vi "CRYOne Quick Lunch Menu.vi"() -> ()   [LabVIEW 2013]
uses:
  CRYMainGlobal.vi
  CRYWindow/SubVI/CRYMain Sub Window Global.vi
panel:
  out "Arrow2":bool
  out "Arrow1":bool
  out "MarkImage":bool
  in  "Show Dialog Prompt":bool caption="Do not show this dialog again"
  out "bReturn":bool
  in  "Calibrate Microphone":bool caption="OK"
  in  "Setup Test":bool caption="OK"
  in  "Self Test":bool caption="OK"
  in  "stop":bool
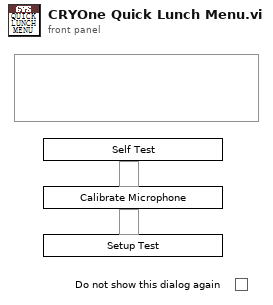
[diagram p1: front panel]
types:
  T1 = enum32{"Invalid", "Standard", "Closed", "Hidden", "Minimized", "Maximized"}
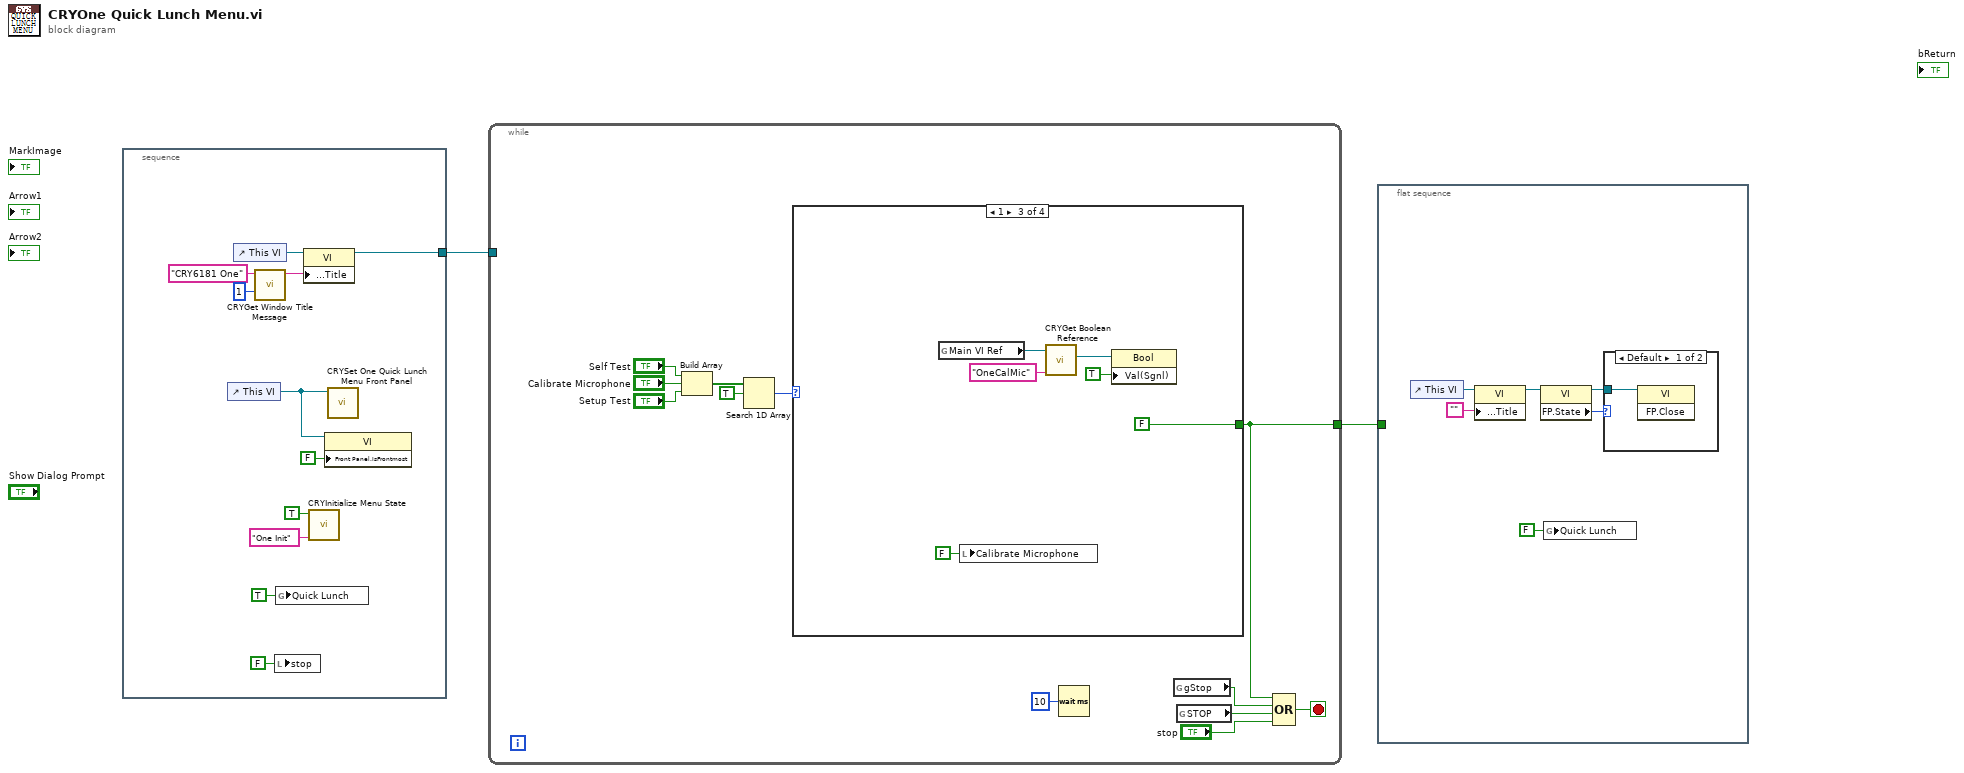
[diagram p0: block diagram]
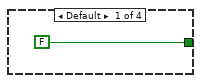
[diagram p3: hidden frame]
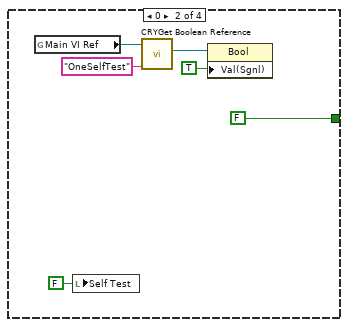
[diagram p4: hidden frame]
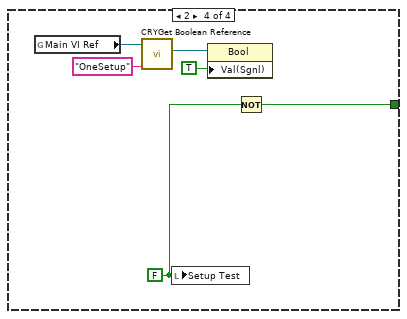
[diagram p5: hidden frame]
diagram:
  n1 = stacked-sequence {
    tunnel: [w6] -> w1
    frame #0 {
      n2 = control-ref of="This VI"() -> (w8:refnum<vi>)
      n3 = control-ref of="This VI"() -> (w11:refnum<vi>)
      n4 = call "CRYGet Window Title Message.vi"("No"=1 ("Error No"), "Kind"="CRY6181 One") -> ("Multibyte String"=w10:string)  [unwired: 4 in, 5 out]
      n5 = local write "stop"(FALSE ("stop")) -> ()
      n6 = global write "CRYMainGlobal.vi" "Quick Lunch"(TRUE ("Quick Lunch")) -> ()
      n7 = property class="VI"(reference=w11, "Front Panel.Title"=w10) -> (reference out=w6:refnum<vi>)  [unwired: 1 in, 1 out]
      n8 = call "CRYInitialize Menu State.vi"("sAction"="One Init", "Is Disable?"=TRUE) -> ()  [unwired: 10 out]
      n9 = property class="VI"(reference=w8, "Front Panel.IsFrontmost"=FALSE ("Front Panel Window:Is Frontmost")) -> ()  [unwired: 1 in, 2 out]
      n10 = call "CRYSet One Quick Lunch Menu Front Panel.vi"("Vi Ref In"=w8) -> ()  [unwired: 10 in, 1 out]
    }
  }
  n11 = while {
    tunnel: [w15] -> w2
    tunnel: w1 -> [_]
    stop <- w14 stop-if-true
    n12 = Build Array("Self Test", "Calibrate Microphone", "Setup Test") -> (w21:bool[])
    n13 = Search 1D Array(1D array=w21, element=TRUE) -> (index of element=w19:i32)  [unwired: 1 in]
    n14 = case shown="1" w19 {
      tunnel: [FALSE FALSE FALSE w43] -> w15
      frame Default {
      }
      frame 0 {
        n15 = global read "CRYMain Sub Window Global.vi" "Main VI Ref"() -> (w30:refnum<vi>)
        n16 = local write "Self Test"(FALSE ("Self Test")) -> ()
        n17 = call "CRYGet Boolean Reference.vi"("Label Name"="OneSelfTest", "VI Refnum"=w30) -> ("Boolean Ref"=w28:refnum<vi>)  [unwired: 7 in, 2 out]
        n18 = property class="Bool"(reference=w28, "Val(Sgnl)"=TRUE) -> ()  [unwired: 1 in, 2 out]
      }
      frame 1 {
        n19 = global read "CRYMain Sub Window Global.vi" "Main VI Ref"() -> (w37:refnum<vi>)
        n20 = local write "Calibrate Microphone"(FALSE ("Calibrate Microphone")) -> ()
        n21 = call "CRYGet Boolean Reference.vi"("Label Name"="OneCalMic", "VI Refnum"=w37) -> ("Boolean Ref"=w35:refnum<vi>)  [unwired: 7 in, 2 out]
        n22 = property class="Bool"(reference=w35, "Val(Sgnl)"=TRUE) -> ()  [unwired: 1 in, 2 out]
      }
      frame 2 {
        w44 = FALSE ("Setup Test")
        n23 = global read "CRYMain Sub Window Global.vi" "Main VI Ref"() -> (w42:refnum<vi>)
        n24 = call "CRYGet Boolean Reference.vi"("Label Name"="OneSetup", "VI Refnum"=w42) -> ("Boolean Ref"=w40:refnum<vi>)  [unwired: 7 in, 2 out]
        n25 = local write "Setup Test"(w44) -> ()
        n26 = property class="Bool"(reference=w40, "Val(Sgnl)"=TRUE) -> ()  [unwired: 1 in, 2 out]
        n27 = Not(x=w44) -> (.not. x?=w43:bool)
      }
    }
    n28 = Wait (ms)(milliseconds to wait=u32 10) -> ()  [unwired: 1 out]
    n29 = global read "CRYMain Sub Window Global.vi" "gStop"() -> (w18:bool)
    n30 = global read "CRYMainGlobal.vi" "STOP"() -> (w16:bool)
    n31 = Compound Arithmetic op=OR(w15, w18, w16, "stop") -> (w14:bool)
  }
  n32 = flat-sequence {
    tunnel: w2 -> [_]
    frame #0 {
      n33 = control-ref of="This VI"() -> (w50:refnum<vi>)
      n34 = property class="VI"(reference=w50, "Front Panel.Title"="") -> (reference out=w48:refnum<vi>)  [unwired: 1 in, 1 out]
      n35 = property class="VI"(reference=w48) -> (reference out=w46:refnum<vi>, "FP.State"=w47:T1)  [unwired: 1 in, 1 out]
      n36 = global write "CRYMainGlobal.vi" "Quick Lunch"(FALSE ("Quick Lunch")) -> ()
      n37 = case shown="Default" w47 {
        tunnel: w46 -> [w51 _]
        frame Default {
          n38 = invoke class="VI" method="FP.Close"(reference=w51) -> ()  [unwired: 2 in, 3 out]
        }
        frame "Closed" {
        }
      }
    }
  }
